vi "Open.vi"(8 "error in (no error)":errorcluster caption="entrée d'erreur (pas d'erreur)", 11 "Process (Default) en entrée":refnum<class "Process (Default).lvclass">) -> (0 "error out":errorcluster caption="sortie d'erreur", 3 "Process (Default) en sortie":refnum<class "Process (Default).lvclass">)   [LabVIEW 2020, in "Library Instrument & Equipement.lvlib" / "Process (Default).lvclass"]
uses:
  Process (Default).lvclass
  Process (Default).lvclass/Process (Default).ctl
  Variable dispatch.vi
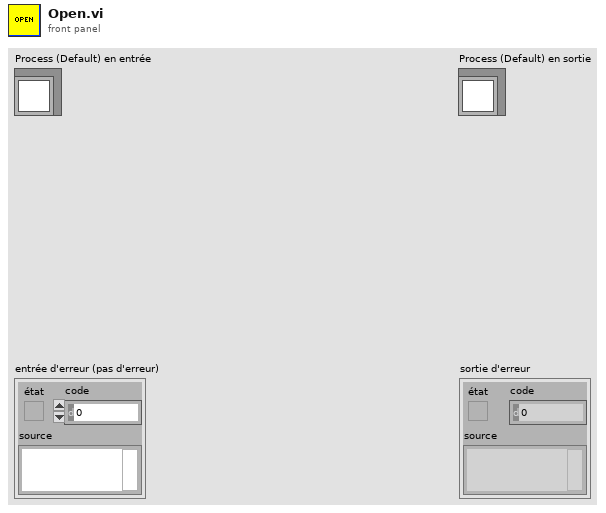
[diagram p1: front panel]
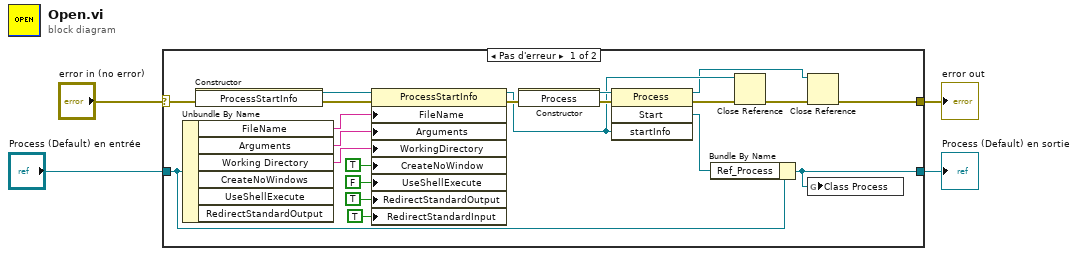
[diagram p0: block diagram]
diagram:
  n1 = case shown="Pas d'erreur" "error in (no error)" {
    selector: "error in (no error)" -> [w10 w27]
    tunnel: [w8 w27] -> w3
    tunnel: [w6 w26] -> w1
    tunnel: "Process (Default) en entrée" -> [w9 w26]
    frame No Error {
      n2 = Unbundle By Name(w9) -> ("FileName"=w19:string, "Arguments"=w17:string, "Working Directory"=w16:string)  [unwired: 3 out]
      n3 = constructor class="ProcessStartInfo"(error in=w10) -> (reference out=w23:refnum<k24>, error out=w11:errorcluster)  [unwired: 2 in, 1 out]
      n4 = property class="ProcessStartInfo"(reference=w23, error in=w11, "FileName"=w19, "Arguments"=w17, "WorkingDirectory"=w16, "CreateNoWindow"=TRUE, "UseShellExecute"=FALSE, "RedirectStandardOutput"=TRUE, "RedirectStandardInput"=TRUE) -> (reference out=w15:refnum<k24>, error out=w20:errorcluster)
      n5 = constructor class="Process"(error in=w20) -> (reference out=w24:refnum<k24>, error out=w25:errorcluster)  [unwired: 2 in, 1 out]
      n6 = invoke class="Process" method="Start"(reference=w24, error in=w25, "startInfo"=w15) -> (reference out=w13:refnum<k24>, error out=w14:errorcluster, "Start"=w7:refnum<k24>)  [unwired: 1 in, 1 out]
      n7 = Bundle By Name(cluster=w9, "Ref_Process"=w7) -> (w6:refnum<class "Process (Default).lvclass">)
      n8 = Close Reference(reference=w15, error in (no error)=w14) -> (error out=w12:errorcluster)
      n9 = Close Reference(reference=w13, error in (no error)=w12) -> (error out=w8:errorcluster)
      n10 = global write "Variable dispatch.vi" "Class Process"(w6) -> ()
    }
    frame Error {
    }
  }
  "error out" <- w3
  "Process (Default) en sortie" <- w1
